vi "Test App Error Handler is Configured as App Process Error Handler for Process Added after Start.vi"(8 "error in (no error)":errorcluster, 11 "Rig Test In":refnum<class "Application Test.lvclass">) -> (0 "error out":errorcluster, 3 "Rig Test Out":refnum<class "Application Test.lvclass">)   [LabVIEW 2020, in "Application Test.lvclass"]
uses:
  Application Test.lvclass
  Framework/Process/Process.lvclass
  Mock Error Handler/Mock Error Handler.lvclass
  <vilib>/Asteme/LUnit/Test Case.lvclass
  Framework/Application/Application.lvclass
  C:/Users/anton/Documents/GitHub/Triarc-Framework/source/Framework/Process/Process.lvclass
  C:/Users/anton/Documents/GitHub/Triarc-Framework/source/Framework/Base/Base.lvclass
  C:/Users/anton/Documents/GitHub/Triarc-Framework/source/Framework/Configuration File/Configuration File.lvclass
  C:/Users/anton/Documents/GitHub/Triarc-Framework/source/Framework/Error Handler Interface/Error Handler Interface.lvclass
  C:/Users/anton/Documents/GitHub/Triarc-Framework/source/Framework/Application/Application.lvclass
  Mock Process/Mock Process.lvclass
  C:/Users/anton/Documents/GitHub/Triarc-Framework/source/Framework Test/Mock Process/Mock Process.lvclass
  C:/Users/anton/Documents/GitHub/Triarc-Framework/source/Framework/Helper Loop/Helper Loop.lvclass
  C:/Users/anton/Documents/GitHub/Triarc-Framework/source/Framework Test/Mock Error Handler/Mock Error Handler.lvclass
  C:/Users/anton/Documents/GitHub/Triarc-Framework/source/Framework Test/Process Test/Process Test.lvclass
  C:/Users/anton/Documents/GitHub/Triarc-Framework/source/Framework Test/Base Class Test/Base Test.lvclass
  C:/Program Files (x86)/National Instruments/LabVIEW 2020/vi.lib/Asteme/LUnit/Test Case.lvclass
  C:/Users/anton/Documents/GitHub/Triarc-Framework/source/Framework Test/Application Test/Application Test.lvclass
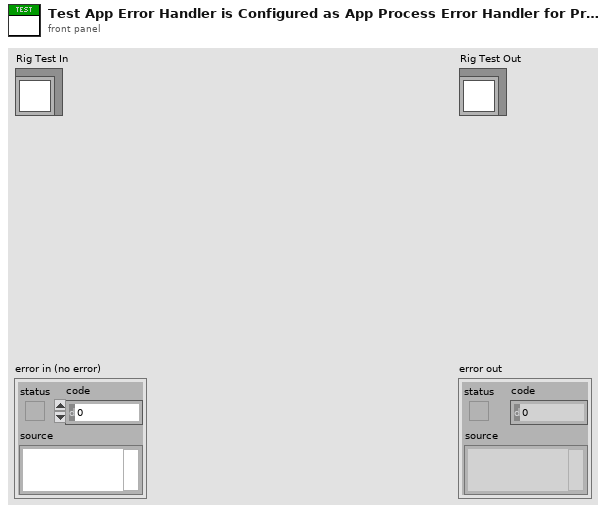
[diagram p1: front panel]
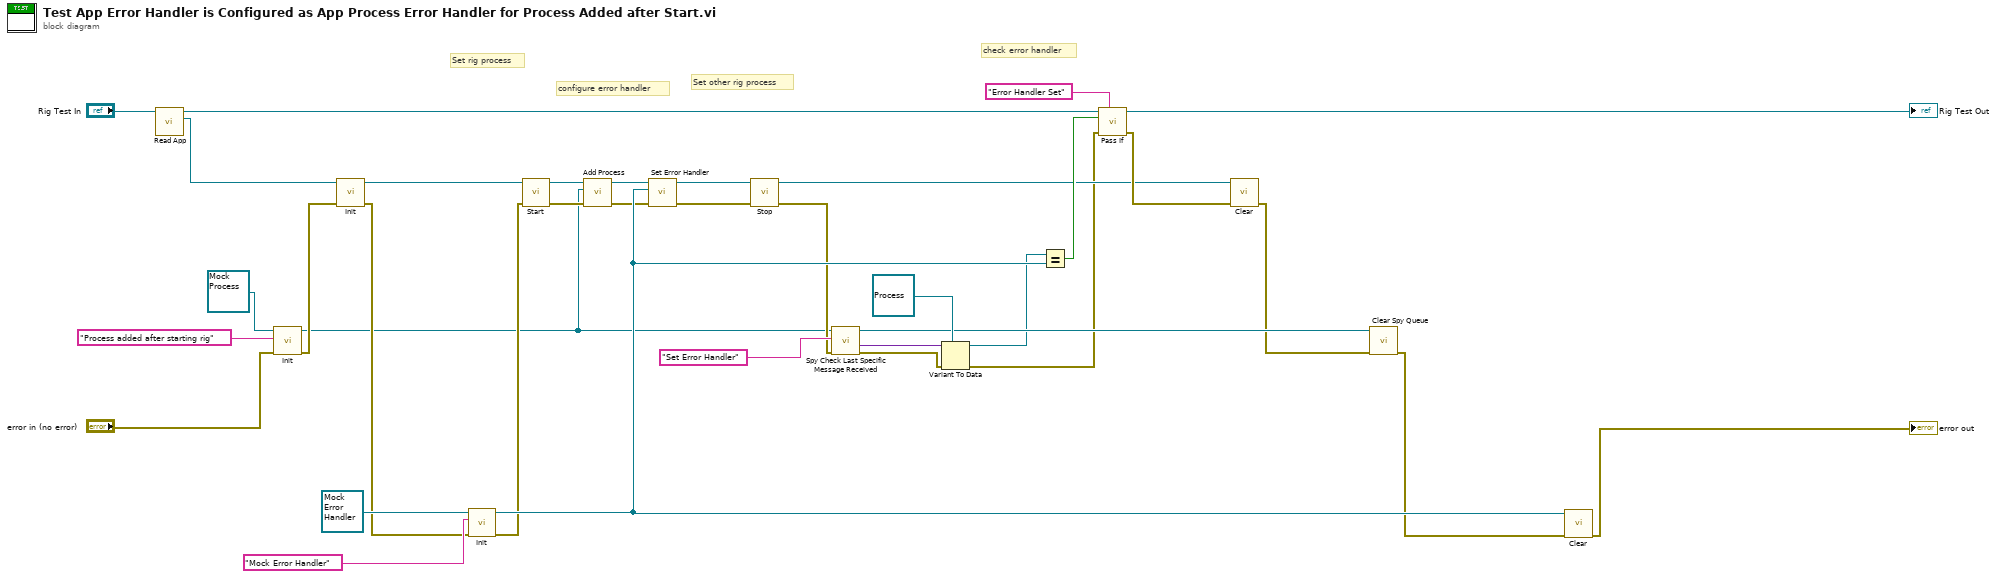
[diagram p0: block diagram]
diagram:
  # "check error handler"
  # "Set other rig process"
  # "configure error handler"
  # "Set rig process"
  n1 = call "Read App.vi"("Application Test In"="Rig Test In") -> ("App out"=w35:refnum<class "Application.lvclass">, "Application Test Out"=w29:refnum<class "Application Test.lvclass">)  [unwired: 8 in, 1 out]
  n2 = call-dynamic "Init.vi"("error in (no error)"="error in (no error)", "Name"="Process added after starting rig", "Mock Process In"=refnum<class "Mock Process.lvclass"> refnum ("Mock Process.lvclass")) -> ("error out"=w21:errorcluster, "Mock Process Out"=w3:refnum<class "Mock Process.lvclass">)  [unwired: 7 in]
  n3 = call-dynamic "Init.vi"("error in (no error)"=w21, "Process In"=w35) -> ("error out"=w20:errorcluster, "Process Out"=w34:refnum<class "Application.lvclass">)  [unwired: 8 in]
  n4 = call-dynamic "Init.vi"("error in (no error)"=w20, "Name"="Mock Error Handler", "Mock Error Handler In"=refnum<class "Mock Error Handler.lvclass"> refnum ("Mock Error Handler.lvclass")) -> ("error out"=w25:errorcluster, "Mock Error Handler Out"=w27:refnum<class "Mock Error Handler.lvclass">)  [unwired: 7 in]
  n5 = call "Start.vi"("error in (no error)"=w25, "Process In"=w34) -> ("error out"=w5:errorcluster, "Process Out"=w7:refnum<class "Application.lvclass">)  [unwired: 8 in]
  n6 = call "Add Process.vi"("error in (no error)"=w5, "Process"=w3, "Rig In"=w7) -> ("error out"=w4:errorcluster, "Rig Out"=w6:refnum<class "Application.lvclass">)  [unwired: 7 in]
  n7 = call "Set Error Handler.vi"("error in (no error)"=w4, "Error Handler"=w27, "Process In"=w6) -> ("error out"=w32:errorcluster, "Process Out"=w33:refnum<class "Application.lvclass">)  [unwired: 7 in]
  n8 = call "Stop.vi"("error in (no error)"=w32, "Process In"=w33) -> ("error out"=w14:errorcluster, "Process Out"=w16:refnum<class "Application.lvclass">)  [unwired: 7 in, 1 out]
  n9 = call "Spy Check Last Specific Message Received.vi"("error in (no error)"=w14, "Specific Call"="Set Error Handler", "Mock Rig Process In"=w3) -> ("error out"=w8:errorcluster, "Message Data"=w13:variant, "Mock Rig Process Out"=w11:refnum<class "Mock Process.lvclass">)  [unwired: 5 in, 1 out]
  n10 = Variant To Data(error in=w8, type=refnum<class "Process.lvclass"> refnum ("Process In"), Variant=w13) -> (data=w10:refnum<class "Process.lvclass">, error out=w9:errorcluster)
  n11 = Equal?(x=w10, y=w27) -> (x = y?=w18:bool)
  n12 = call <vilib>:"Pass If.vi"("Description"="Error Handler Set", "error in (no error)"=w9, "Pass?"=w18, "Test Case In"=w29) -> ("error out"=w19:errorcluster, "Test Case Out"=→"Rig Test Out":refnum<class "Application Test.lvclass">)  [unwired: 6 in]
  n13 = call-dynamic "Clear.vi"("error in (no error)"=w19, "Application In"=w16) -> ("error out"=w2:errorcluster)  [unwired: 8 in, 1 out]
  n14 = call-dynamic "Clear Spy Queue.vi"("error in (no error)"=w2, "Mock Process In"=w11) -> ("error out"=w1:errorcluster)  [unwired: 8 in, 1 out]
  n15 = call-dynamic "Clear.vi"("error in (no error)"=w1, "Process In"=w27) -> ("error out"=→"error out":errorcluster)  [unwired: 8 in, 1 out]
